vi "4-7.vi"() -> (0 "猜测次数":i32, 1 "随机的数":i32)   [LabVIEW 2017]
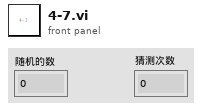
[diagram p1: front panel]
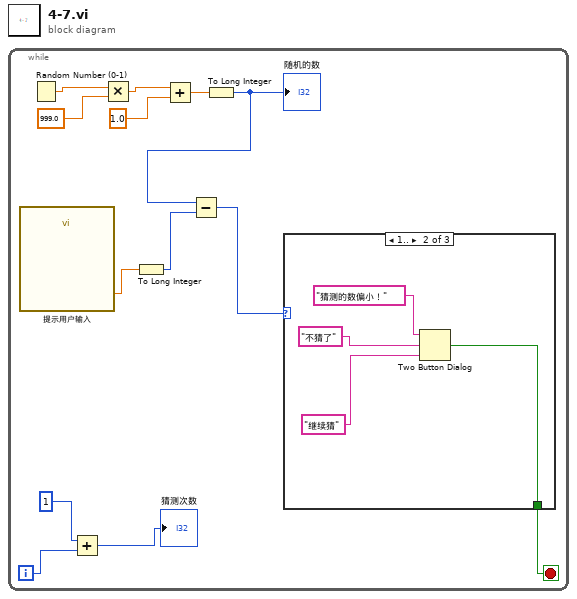
[diagram p0: block diagram]
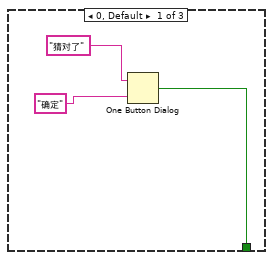
[diagram p2: hidden frame]
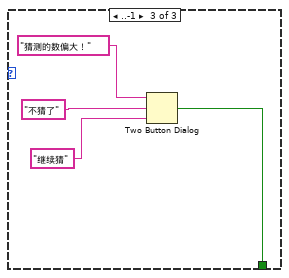
[diagram p3: hidden frame]
diagram:
  n1 = while {
    i -> [w1]
    stop <- w4 stop-if-true
    n2 = call "提示用户输入"() -> ("请在1-1000猜"=w6:dbl)  [unwired: 17 in, 2 out]
    n3 = Random Number (0-1)() -> (number: 0 to 1=w13:dbl)
    n4 = Add(x=1, y=w1) -> (x+y=→"猜测次数":i32)
    n5 = Multiply(x=w13, y=999.0) -> (x*y=w11:dbl)
    n6 = To Long Integer(number=w6) -> (32bit integer=w5:i32)
    n7 = Add(x=w11, y=1.0) -> (x+y=w9:dbl)
    n8 = To Long Integer(number=w9) -> (32bit integer=w8:i32)
    "随机的数" <- w8
    n9 = Subtract(x=w8, y=w5) -> (x-y=w7:i32)
    n10 = case shown="1.." w7 {
      tunnel: [w14 w17 w21] -> w4
      frame 0, Default {
        n11 = One Button Dialog(message="猜对了", button name ("OK")="确定") -> (true=w14:bool)
      }
      frame 1.. {
        n12 = Two Button Dialog(message="猜测的数偏小！", 1:"继续猜", 2:"不猜了") -> (T button?=w17:bool)
      }
      frame ..-1 {
        n13 = Two Button Dialog(message="猜测的数偏大！", 1:"继续猜", 2:"不猜了") -> (T button?=w21:bool)
      }
    }
  }
